vi "AskVersion.vi"(8 "error in":errorcluster, 11 "VISA Refnum in":refnum<visa-resource-name>) -> (0 "error out":errorcluster, 2 "Version":string, 3 "VISA Refnum out":refnum<visa-resource-name>)   [LabVIEW 2017]
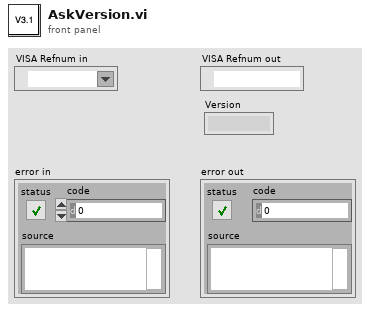
[diagram p1: front panel]
types:
  T1 = enum16{"big-endian, network order", "native, host order", "little-endian"}
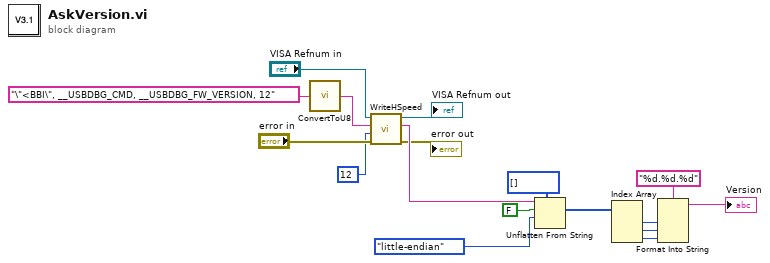
[diagram p0: block diagram]
diagram:
  n1 = call <userlib>:"ConvertToU8.vi"("struct"="\"<BBI\", __USBDBG_CMD, __USBDBG_FW_VERSION, 12" ("write buffer")) -> ("Binary"=w3:string)
  n2 = call <userlib>:"WriteHSpeed.vi"("error in"="error in", "Reply length"=12 ("Reply"), "write buffer"=w3, "VISA Refnum in"="VISA Refnum in") -> ("error out"=→"error out":errorcluster, "read buffer"=w13:string, "VISA Refnum out"=→"VISA Refnum out":refnum<visa-resource-name>)  [unwired: 5 in]
  n3 = Unflatten From String(type=i32[] [], binary string=w13, data includes array or string size? (T)=FALSE ("prepend array or string size? (T)"), byte order (0:big-endian, network order)=T1."little-endian") -> (value=w10:i32[])  [unwired: 1 in, 2 out]
  n4 = Index Array(array=w10) -> (element #1=w9:i32, element #2=w7:i32, element #3=w6:i32)  [unwired: 3 in]
  n5 = Format Into String(format string="%d.%d.%d", w9, w7, w6) -> (resulting string=→"Version":string)  [unwired: 2 in, 1 out]
